vi "NOYITO-2Channel_MAIN.vi"(8 "error in (no error)":errorcluster, 11 "RelayControlHexCMD":T1(ring)) -> (0 "error out":errorcluster, 2 "RelayResponse":string, 3 "Success":bool)   [LabVIEW 2020, in "NOYITO 2 Channel Relay Driver.lvlib"]
doc: "Developed By: J Branch\nLast Update: 10/9/2022\n\nDescription: Allows user control of the NOYITO 2 channel relay module through LabVIEW. This relay module is a simple to use, low-cost, of the shelf serial controlled dual SPDT relay module.\n\nSee the Device Desc tab to view more about the device description."
uses:
  NOYITO 2 Channel Relay Driver.lvlib
panel:
  in  "Tab Control":enum32{"Front", "Error Clusters", "Device Desc"}(tab)
  out "Device Description":string
  # "OPEN --> Turns Relay \"ON\"\nLED should be lit above relay when OPEN\nCLOSED --> Turns Relay \"OFF\"\n\nOPEN refers to COM connected to NO\nCLOSED refers to COM connected to NC"
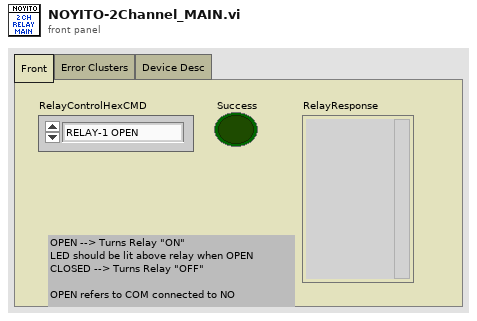
[diagram p1: front panel]
types:
  T1 = enum16{"RELAY-1 OPEN", "RELAY-1 CLOSED", "RELAY-2 OPEN", "RELAY-2 CLOSED", "GET RELAY STATUS"}
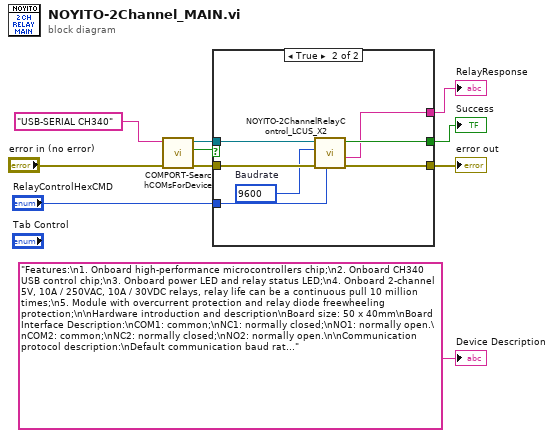
[diagram p0: block diagram]
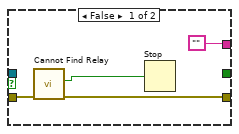
[diagram p2: hidden frame]
diagram:
  n1 = call "COMPORT-SearchCOMsForDevice.vi"("error in (no error)"="error in (no error)", "SearchSTR"="USB-SERIAL CH340") -> ("error out"=w9:errorcluster, "Device COM found?"=w6:bool, "COM-out"=w10:refnum<visa-resource-name>)  [unwired: 7 in]
  n2 = case shown="True" w6 {
    tunnel: w10 -> [_ w21]
    tunnel: w9 -> [w13 w20]
    tunnel: "RelayControlHexCMD" -> [_ w19]
    tunnel: [w12 w18] -> w4
    tunnel: [_ w17] -> w3
    tunnel: ["" w15] -> w2
    frame False {
      n3 = call "Cannot Find Relay"("error in (no error)"=w13) -> ("error out"=w12:errorcluster, "OK"=w11:bool)  [unwired: 9 in]
      n4 = Stop(stop? (T)=w11) -> ()
    }
    frame True {
      w16 = u32 9600 items=["4800"=4800, "9600"=9600, "19200"=19200, "38400"=38400, "57600"=57600]  # Baudrate
      n5 = call "NOYITO-2ChannelRelayControl_LCUS_X2.vi"("RelayControlHexCMD"=w19, "error in (no error)"=w20, "Baudrate"=w16, "NOYITO-2CH COM"=w21) -> ("error out"=w18:errorcluster, "RelayResponse"=w15:string, "Success"=w17:bool)  [unwired: 5 in]
    }
  }
  "error out" <- w4
  "Success" <- w3
  "RelayResponse" <- w2
  "Device Description" <- "Features:\n1. Onboard high-performance microcontrollers chip;\n2. Onboard CH340 USB control chip;\n3. Onboard power LED and relay status LED;\n4. Onboard 2-channel 5V, 10A / 250VAC, 10A / 30VDC relays, relay life can be a continuous pull 10 million times;\n5. Module with overcurrent protection and relay diode freewheeling protection;\n\nHardware introduction and description\nBoard size: 50 x 40mm\nBoard Interface Description:\nCOM1: common;\nNC1: normally closed;\nNO1: normally open.\nCOM2: common;\nNC2: normally closed;\nNO2: normally open.\n\nCommunication protocol description:\nDefault communication baud rate: 9600BPS\nTurn on the 1-channel relay switch: A0 01 01 A2\nTurn off the 1-channel relay switch: A0 01 00 A1\nTurn on the 2-channel relay switch: A0 02 01 A3\nTurn off the 2-channel relay switch: A0 02 00 A2\n\nUSB switch communication protocol\nData (1)start flag (default is 0xA0)\nData (2) switch address codes (0x01 and 0x02 represent the first and second switches, respectively)\nData (3) operating data (0x00 is \"off\", 0x01 is \"on\")\nData (4) check code\n\nUsage Description:\n1. Connect the USB relay module to the computer and install the CH340 USB to serial chip driver\n2. Open the STC-ISP, SSCOM32 such serial debugging software, select the baud rate of 9600, in hexadecimal (hex) form send A0 01 01 A2 and A0 02 01 A3 can be opened the first and second relay ; Send in hexadecimal (hex) A0 01 00 A1 and A0 02 00 A2 can be turned off the first and second relay, respectively." ("Device Description")
